vi "TwTpsGetLastSetValue.vi"(2 "moduleCode":i32, 3 "error in (no error)":errorcluster) -> (0 "value":dbl, 1 "error out":errorcluster)   [LabVIEW 2009]
uses:
  TofDaqDll.dll
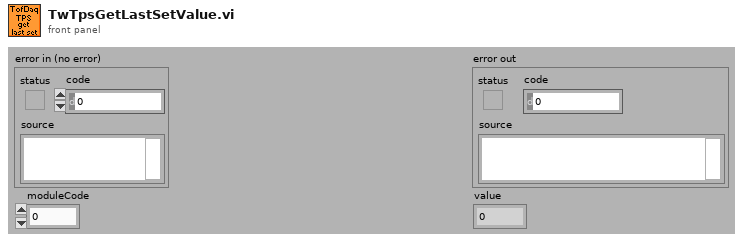
[diagram p1: front panel]
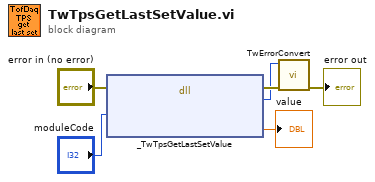
[diagram p0: block diagram]
diagram:
  n1 = dll-call lib="C:/src/TofDaq/APIandWrappers/LabView/TofDaqDll/TofDaqDll.dll" fn="_TwTpsGetLastSetValue"(error in="error in (no error)", "moduleCode"="moduleCode") -> (error out=w5:errorcluster, "TwRetVal"=w3:i32, "value"=→"value":dbl)  [unwired: 3 in, 2 out]
  n2 = call "TwErrorConvert.vi"("error in (no error)"=w5, "error code"=w3) -> ("error out"=→"error out":errorcluster)  [unwired: 9 out]
